vi "测量数据区.vi"(11 "数组":u16[](array[numeric]) format="%04xH") -> (3 "测量数据区":T1 {"单位" items=["ug/L", "mg/L", "ppm", "mg/m3", "cm", "ppb", "ug/m3", "%", "nmol/mol", "umol/mol", "MPN/L", "MPN/100ml", "ng/m3", "NTU", "无量纲", "ms/cm", "us/cm", "℃", "mV", "万个/L"]})   [LabVIEW 2022 SP3, in "斯坦道通用流路CODmn.lvlib"]
uses:
  <vilib>/Utility/miscctls.llb/LVDateTimeRec.ctl
panel:
  # "共占用105 WORD"
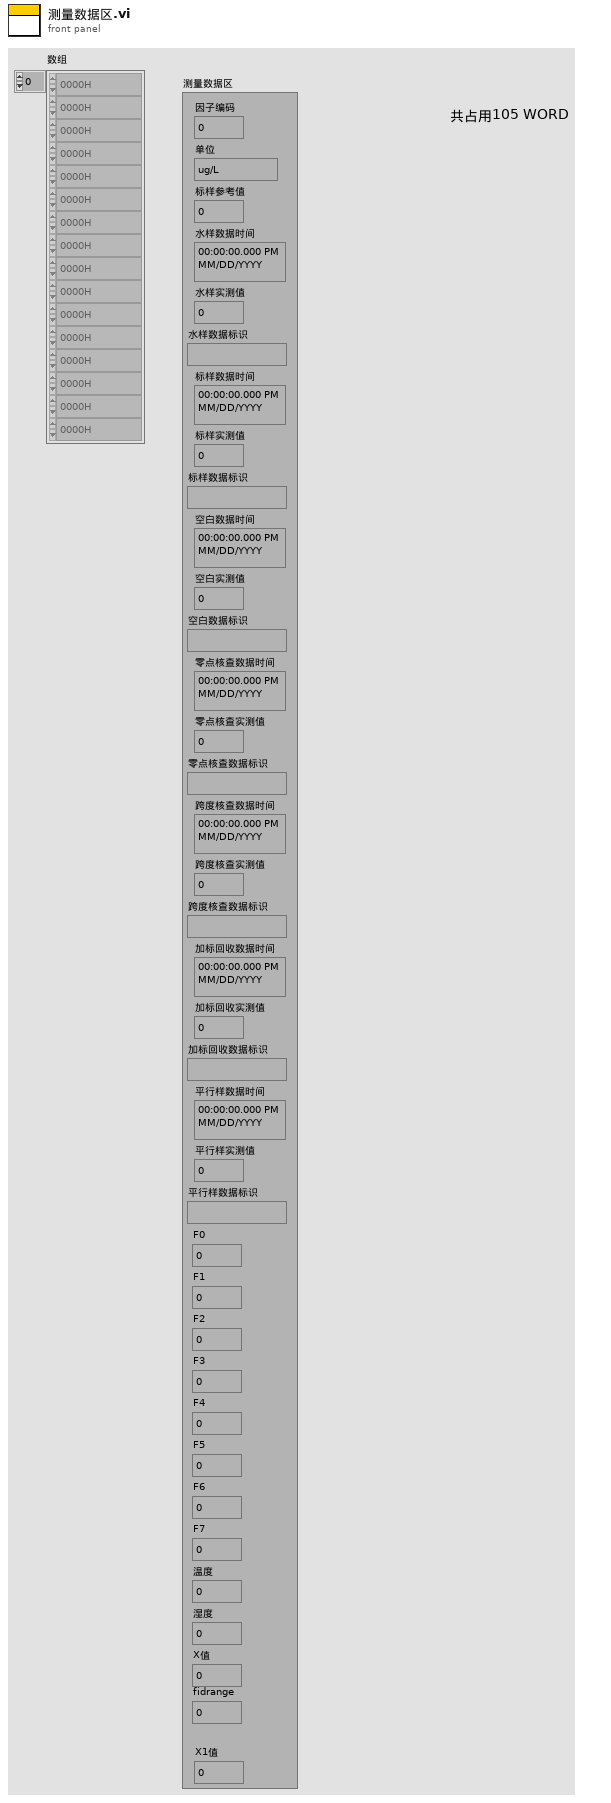
[diagram p1: front panel]
types:
  T1 = cluster{"因子编码":u32, "单位":u16, "标样参考值":sgl, "水样数据时间":timestamp, "水样实测值":sgl, "水样数据标识":string, "标样数据时间":timestamp, "标样实测值":sgl, "标样数据标识":string, "空白数据时间":timestamp, "空白实测值":sgl, "空白数据标识":string, "零点核查数据时间":timestamp, "零点核查实测值":sgl, "零点核查数据标识":string, "跨度核查数据时间":timestamp, "跨度核查实测值":sgl, "跨度核查数据标识":string, "加标回收数据时间":timestamp, "加标回收实测值":sgl, "加标回收数据标识":string, "平行样数据时间":timestamp, "平行样实测值":sgl, "平行样数据标识":string, "F0":sgl, "F1":sgl, "F2":sgl, "F3":sgl, "F4":sgl, "F5":sgl, "F6":sgl, "F7":sgl, "温度":sgl, "湿度":sgl, "X值":sgl, "fidrange":u16, "X1值":sgl}
  T2 = typedef "LVDateTimeRec.ctl" = cluster{"fractional second":dbl, "second":i32, "minute":i32, "hour":i32, "day of month":i32, "month":i32, "year":i32, "day of week":i32, "day of year":i32, "DST":i32}
  T3 = cluster{u32, u16, sgl, "time stamp":timestamp, sgl, string, "time stamp":timestamp, sgl, string, "time stamp":timestamp, sgl, string, "time stamp":timestamp, sgl, string, "time stamp":timestamp, sgl, string, "time stamp":timestamp, sgl, string, "time stamp":timestamp, sgl, string, sgl, sgl, sgl, sgl, sgl, sgl, sgl, sgl, sgl, sgl, sgl, "数值":u16, sgl}
  T4 = cluster{"DWORD":i32, "WORD":u16, "FLOAT":sgl, "time stamp":timestamp, "数值":sgl, "string":string, "time stamp":timestamp, "数值":sgl, "string":string, "time stamp":timestamp, "数值":sgl, "string":string, "time stamp":timestamp, "数值":sgl, "string":string, "time stamp":timestamp, "数值":sgl, "string":string, "time stamp":timestamp, "数值":sgl, "string":string, "time stamp":timestamp, "数值":sgl, "string":string, "FLOAT":sgl, "FLOAT":sgl, "FLOAT":sgl, "FLOAT":sgl, "FLOAT":sgl, "FLOAT":sgl, "FLOAT":sgl, "FLOAT":sgl, "FLOAT":sgl, "FLOAT":sgl, "FLOAT":sgl, "数值":u16, "FLOAT":sgl}
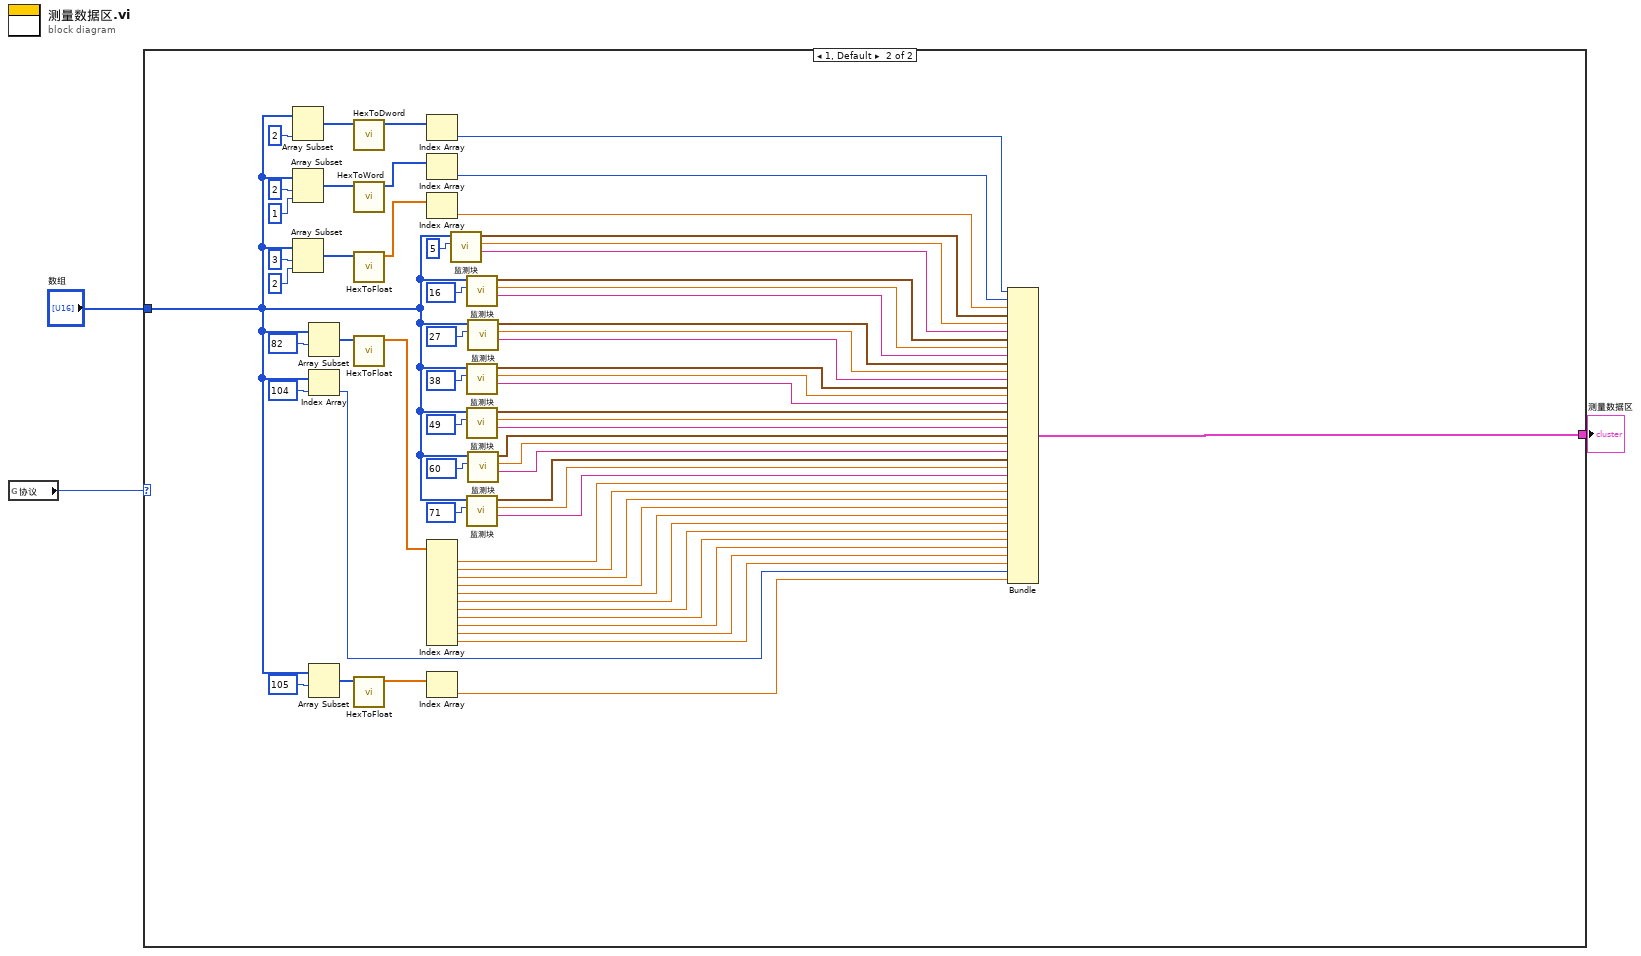
[diagram p0: block diagram]
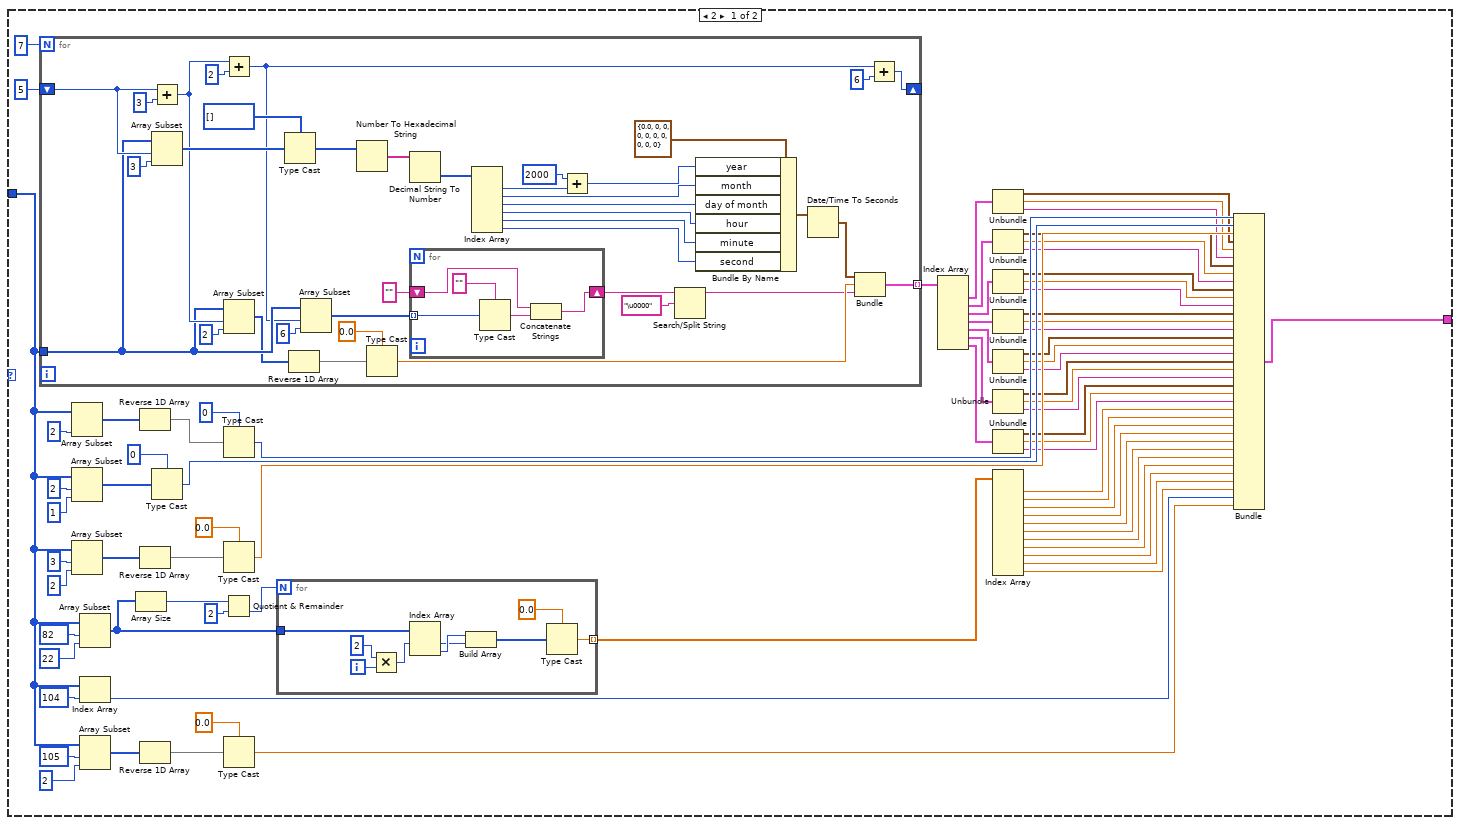
[diagram p2: hidden frame]
diagram:
  n1 = global read "总磷总氮断电保存全局变量.vi" "协议"() -> (w1:u16)
  n2 = case shown="1, Default" w1 {
    tunnel: [w4 w151] -> w3
    tunnel: "数组" -> [w5 w130]
    frame 2 {
      n3 = for {
        N: 7 -> [_]
        tunnel: w5 -> [w101]
        shift-right: [w90] -> _
        shift-left: 5 ("索引") -> [w108]
        tunnel: [w93] -> w45 mode=indexing
        n4 = Add(x=w108, y=3) -> (x+y=w104:i32)
        n5 = Array Subset(array=w101, index=w108, length=3 ("索引")) -> (w114:u16[])
        n6 = Add(x=w104, y=2) -> (x+y=w92:i32)
        n7 = Array Subset(array=w101, index=w104, length=2 ("长度")) -> (w89:u16[])
        n8 = Type Cast(type=u8[] [], x=w114) -> (*(type *) &x=w116:u8[])
        n9 = Reverse 1D Array(array=w89) -> (reversed array=w88:u16[])
        n10 = Array Subset(array=w101, index=w92, length=6 ("长度")) -> (w97:u16[])
        n11 = Number To Hexadecimal String(2:w116) -> (0:w115:string[])  [unwired: 1 in]
        n12 = Type Cast(type=sgl 0.0, x=w88) -> (*(type *) &x=w95:sgl)
        n13 = Decimal String To Number(string=w115) -> (number=w113:i32[])  [unwired: 2 in, 1 out]
        n14 = for {
          shift-right: [w129] -> w99
          shift-left: "" -> [w126]
          tunnel: w97 -> [w128] mode=indexing
          n15 = Type Cast(type="", x=w128) -> (*(type *) &x=w125:string)
          n16 = Concatenate Strings(w126, w125) -> (w129:string)
        }
        n17 = Index Array(array=w113) -> (element #1=w111:i32, element #2=w121:i32, element #3=w120:i32, element #4=w119:i32, element #5=w118:i32, element #6=w109:i32)  [unwired: 6 in]
        n18 = Add(x=2000 ("y"), y=w111) -> (x+y=w110:i32)
        n19 = Search/Split String(string=w99, search string/char (-)="\u0000" ("搜索字符串")) -> (substring before match=w94:string)  [unwired: 1 in, 2 out]
        n20 = Bundle By Name(cluster=T2 {"fractional second"=0.0, "second"=0, "minute"=0, "hour"=0, "day of month"=0, "month"=0, "year"=0, "day of week"=0, "day of year"=0, "DST"=0} ("日期时间记录"), "year"=w110, "month"=w121, "day of month"=w120, "hour"=w119, "minute"=w118, "second"=w109) -> (w117:T2)
        n21 = Date/Time To Seconds(2:w117) -> (0:w96:timestamp)  [unwired: 1 in]
        n22 = Bundle("time stamp"=w96, w95, w94) -> (w93:cluster{"time stamp":timestamp, sgl, string})  [unwired: 1 in]
        n23 = Add(x=w92, y=6) -> (x+y=w90:i32)
      }
      n24 = Array Subset(array=w5, length=u32 2 ("长度")) -> (w15:u16[])  [unwired: 1 in]
      n25 = Array Subset(array=w5, index=2 ("索引"), length=1 ("长度")) -> (w55:u16[])
      n26 = Array Subset(array=w5, index=3 ("索引"), length=2 ("长度")) -> (w14:u16[])
      n27 = Array Subset(array=w5, index=82 ("索引"), length=22 ("长度")) -> (w12:u16[])
      n28 = Index Array(array=w5, index=104 ("索引")) -> (element=w60:u16)
      n29 = Array Subset(array=w5, index=105 ("索引"), length=2 ("长度")) -> (w7:u16[])
      n30 = Array Size(array=w12) -> (size(s)=w11:i32)
      n31 = Reverse 1D Array(array=w15) -> (reversed array=w16:u16[])
      n32 = Reverse 1D Array(array=w14) -> (reversed array=w13:u16[])
      n33 = Reverse 1D Array(array=w7) -> (reversed array=w6:u16[])
      n34 = Type Cast(type=u16 0, x=w55) -> (*(type *) &x=w54:u16)
      n35 = Type Cast(type=u32 0, x=w16) -> (*(type *) &x=w57:u32)
      n36 = Type Cast(type=sgl 0.0, x=w13) -> (*(type *) &x=w50:sgl)
      n37 = Quotient & Remainder(x=w11, y=2) -> (floor(x/y)=w9:i32)  [unwired: 1 out]
      n38 = Type Cast(type=sgl 0.0, x=w6) -> (*(type *) &x=w46:sgl)
      n39 = for {
        N: w9 -> [_]
        tunnel: w12 -> [w87]
        tunnel: [w79] -> w8 mode=indexing
        i -> [w86]
        n40 = Multiply(x=2, y=w86) -> (x*y=w84:i32)
        n41 = Index Array(array=w87, index #1=w84) -> (element #1=w82:u16, element #2=w83:u16)  [unwired: 1 in]
        n42 = Build Array(w83, w82) -> (w81:u16[])
        n43 = Type Cast(type=sgl 0.0, x=w81) -> (*(type *) &x=w79:sgl)
      }
      n44 = Index Array(array=w45) -> (element #1=w44:cluster{"time stamp":timestamp, sgl, string}, element #2=w43:cluster{"time stamp":timestamp, sgl, string}, element #3=w42:cluster{"time stamp":timestamp, sgl, string}, element #4=w41:cluster{"time stamp":timestamp, sgl, string}, element #5=w40:cluster{"time stamp":timestamp, sgl, string}, element #6=w39:cluster{"time stamp":timestamp, sgl, string}, element #7=w38:cluster{"time stamp":timestamp, sgl, string})  [unwired: 7 in]
      n45 = Unbundle(w44) -> ("time stamp"=w37:timestamp, w36:sgl, w35:string)
      n46 = Unbundle(w43) -> ("time stamp"=w34:timestamp, w33:sgl, w32:string)
      n47 = Unbundle(w42) -> ("time stamp"=w31:timestamp, w30:sgl, w29:string)
      n48 = Unbundle(w41) -> ("time stamp"=w28:timestamp, w27:sgl, w26:string)
      n49 = Unbundle(w40) -> ("time stamp"=w25:timestamp, w24:sgl, w23:string)
      n50 = Unbundle(w39) -> ("time stamp"=w22:timestamp, w21:sgl, w20:string)
      n51 = Unbundle(w38) -> ("time stamp"=w19:timestamp, w18:sgl, w17:string)
      n52 = Index Array(array=w8) -> (element #1=w72:sgl, element #2=w71:sgl, element #3=w70:sgl, element #4=w69:sgl, element #5=w68:sgl, element #6=w67:sgl, element #7=w66:sgl, element #8=w65:sgl, element #9=w64:sgl, element #10=w63:sgl, element #11=w62:sgl)  [unwired: 11 in]
      n53 = Bundle(w57, w54, w50, "time stamp"=w37, w36, w35, "time stamp"=w34, w33, w32, "time stamp"=w31, w30, w29, "time stamp"=w28, w27, w26, "time stamp"=w25, w24, w23, "time stamp"=w22, w21, w20, "time stamp"=w19, w18, w17, w72, w71, w70, w69, w68, w67, w66, w65, w64, w63, w62, "数值"=w60, w46) -> (w4:T3)  [unwired: 1 in]
    }
    frame 1, Default {
      n54 = Array Subset(array=w130, length=2 ("长度")) -> (w193:u16[])  [unwired: 1 in]
      n55 = Array Subset(array=w130, index=2 ("索引"), length=1 ("长度")) -> (w188:u16[])
      n56 = Array Subset(array=w130, index=3 ("索引"), length=2 ("长度")) -> (w183:u16[])
      n57 = Array Subset(array=w130, index=82 ("索引")) -> (w149:u16[])  [unwired: 1 in]
      n58 = Index Array(array=w130, index=104 ("索引")) -> (element=w135:u16)
      n59 = Array Subset(array=w130, index=105 ("索引")) -> (w133:u16[])  [unwired: 1 in]
      n60 = call "HexToDword.vi"("数组"=w193) -> ("DWORD"=w191:i32[])  [unwired: 10 in]
      n61 = call "HexToWord.vi"("数组"=w188) -> ("WORD"=w187:u16[])  [unwired: 10 in]
      n62 = call "HexToFloat.vi"("数组"=w183) -> ("FLOAT"=w182:sgl[])  [unwired: 10 in]
      n63 = call "HexToFloat.vi"("数组"=w149) -> ("FLOAT"=w148:sgl[])  [unwired: 10 in]
      n64 = call "HexToFloat.vi"("数组"=w133) -> ("FLOAT"=w132:sgl[])  [unwired: 10 in]
      n65 = Index Array(array=w191) -> (element=w152:i32)  [unwired: 1 in]
      n66 = Index Array(array=w187) -> (element=w186:u16)  [unwired: 1 in]
      n67 = Index Array(array=w182) -> (element=w181:sgl)  [unwired: 1 in]
      n68 = Index Array(array=w148) -> (element #1=w147:sgl, element #2=w146:sgl, element #3=w145:sgl, element #4=w144:sgl, element #5=w143:sgl, element #6=w142:sgl, element #7=w141:sgl, element #8=w140:sgl, element #9=w139:sgl, element #10=w138:sgl, element #11=w137:sgl)  [unwired: 11 in]
      n69 = Index Array(array=w132) -> (element=w131:sgl)  [unwired: 1 in]
      n70 = call "监测块.vi"("索引"=5, "数组"=w130) -> ("string"=w178:string, "数值"=w179:sgl, "time stamp"=w180:timestamp)  [unwired: 7 in]
      n71 = call "监测块.vi"("索引"=16, "数组"=w130) -> ("string"=w173:string, "数值"=w174:sgl, "time stamp"=w175:timestamp)  [unwired: 7 in]
      n72 = call "监测块.vi"("索引"=38, "数组"=w130) -> ("string"=w165:string, "数值"=w166:sgl, "time stamp"=w167:timestamp)  [unwired: 7 in]
      n73 = call "监测块.vi"("索引"=49, "数组"=w130) -> ("string"=w161:string, "数值"=w162:sgl, "time stamp"=w163:timestamp)  [unwired: 7 in]
      n74 = call "监测块.vi"("索引"=71, "数组"=w130) -> ("string"=w153:string, "数值"=w154:sgl, "time stamp"=w155:timestamp)  [unwired: 7 in]
      n75 = call "监测块.vi"("索引"=27, "数组"=w130) -> ("string"=w169:string, "数值"=w170:sgl, "time stamp"=w171:timestamp)  [unwired: 7 in]
      n76 = call "监测块.vi"("索引"=60, "数组"=w130) -> ("string"=w157:string, "数值"=w158:sgl, "time stamp"=w159:timestamp)  [unwired: 7 in]
      n77 = Bundle("DWORD"=w152, "WORD"=w186, "FLOAT"=w181, "time stamp"=w180, "数值"=w179, "string"=w178, "time stamp"=w175, "数值"=w174, "string"=w173, "time stamp"=w171, "数值"=w170, "string"=w169, "time stamp"=w167, "数值"=w166, "string"=w165, "time stamp"=w163, "数值"=w162, "string"=w161, "time stamp"=w159, "数值"=w158, "string"=w157, "time stamp"=w155, "数值"=w154, "string"=w153, "FLOAT"=w147, "FLOAT"=w146, "FLOAT"=w145, "FLOAT"=w144, "FLOAT"=w143, "FLOAT"=w142, "FLOAT"=w141, "FLOAT"=w140, "FLOAT"=w139, "FLOAT"=w138, "FLOAT"=w137, "数值"=w135, "FLOAT"=w131) -> (w151:T4)  [unwired: 1 in]
    }
  }
  "测量数据区" <- w3
